vi "Node Main Operation.vi"(8 "error in (no error)":errorcluster, 11 "Node Actor in":refnum<class "Node Actor.lvclass">) -> (0 "error out":errorcluster, 3 "Node Actor out":refnum<class "Node Actor.lvclass">)   [LabVIEW 2024, in "Node Actor.lvclass"]
uses:
  Node Actor.lvclass
  Message/Message.lvclass/Message.ctl
  Node Actor.lvclass/Node Actor.ctl
  Message/Public Data/Read CMD Type.vi
  Message/Message.lvclass
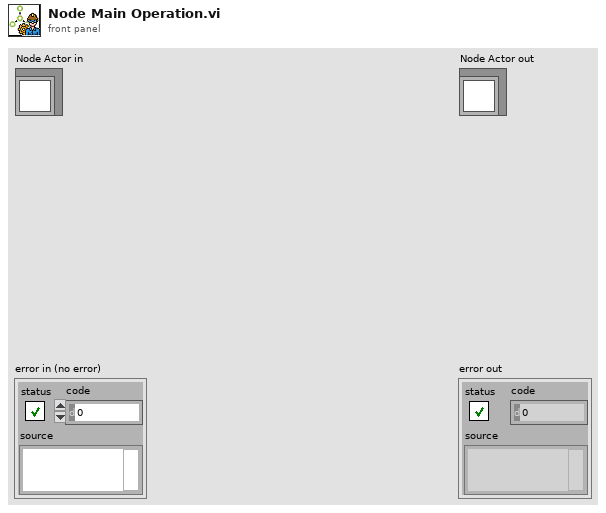
[diagram p1: front panel]
types:
  T1 = typedef "CMD Type.ctl" = enum16{"None", "General CMD", "1st CMD", "2nd CMD", "3rd CMD", "4th CMD", "5th CMD", "6th CMD", "7th CMD"}
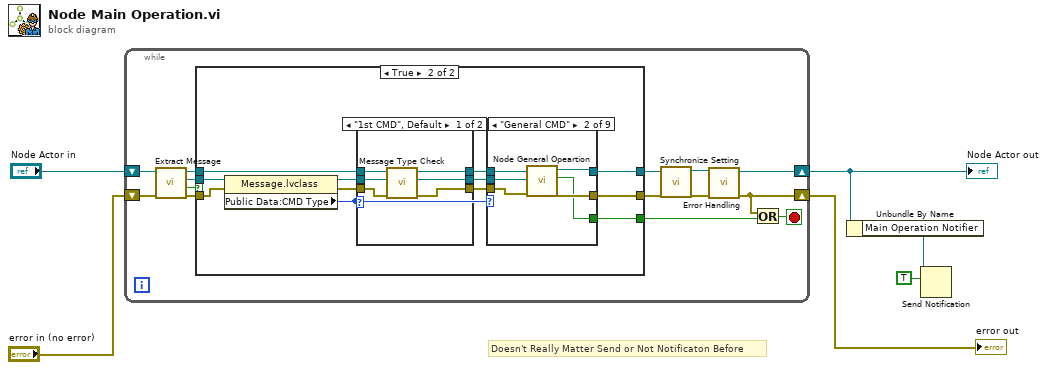
[diagram p0: block diagram]
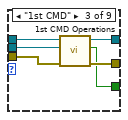
[diagram p5: hidden frame]
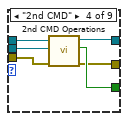
[diagram p6: hidden frame]
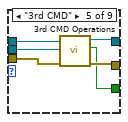
[diagram p7: hidden frame]
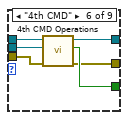
[diagram p8: hidden frame]
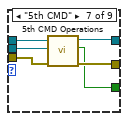
[diagram p9: hidden frame]
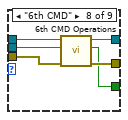
[diagram p10: hidden frame]
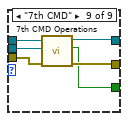
[diagram p11: hidden frame]
diagram:
  # "Doesn't Really Matter Send or Not Notificaton Before"
  n1 = while {
    shift-right: [w12] -> w1
    shift-left: "Node Actor in" -> [w19]
    shift-right: [w11] -> w4
    shift-left: "error in (no error)" -> [w18]
    stop <- w20 stop-if-true
    n2 = call-dynamic "Extract Message.vi"("error in (no error)"=w18, "Node Actor in"=w19) -> ("error out"=w15:errorcluster, "Valid"=w13:bool, "Message Out"=w16:refnum<class "Message.lvclass">, "Node Actor out"=w17:refnum<class "Node Actor.lvclass">)  [unwired: 6 in]
    n3 = case shown="True" w13 {
      tunnel: [w21 w34] -> w8
      tunnel: w17 -> [w22 w26]
      tunnel: w16 -> [_ w31]
      tunnel: w15 -> [w21 w30]
      tunnel: [w22 w33] -> w10
      tunnel: [_ w32] -> w14
      frame False {
      }
      frame True {
        n4 = property class="Message.lvclass"(reference=w31, error in=w30) -> (reference out=w28:refnum<class "Message.lvclass">, error out=w27:errorcluster, "Public Data:CMD Type"=w29:T1)
        n5 = case shown="\"1st CMD\", Default" w29 {
          tunnel: w28 -> [w39 w42]
          tunnel: w27 -> [w38 w41]
          tunnel: w26 -> [w40 w43]
          tunnel: [w35 w43] -> w25
          tunnel: [w36 w42] -> w24
          tunnel: [w37 w41] -> w23
          frame "1st CMD", Default {
            n6 = call-dynamic "Message Type Check.vi"("error in (no error)"=w38, "Message In"=w39, "Node Actor in"=w40) -> ("error out"=w37:errorcluster, "Message Out"=w36:refnum<class "Message.lvclass">, "Node Actor out"=w35:refnum<class "Node Actor.lvclass">)  [unwired: 6 in]
          }
          frame "General CMD" {
          }
        }
        n7 = case shown="\"General CMD\"" w29 {
          tunnel: w24 -> [_ w50 w56 w59 w68 w74 w80 w86 w92]
          tunnel: w25 -> [w45 w51 w57 w63 w69 w75 w81 w87 w93]
          tunnel: [w45 w47 w53 w62 w65 w72 w77 w84 w89] -> w33
          tunnel: w23 -> [w44 w49 w55 w58 w67 w73 w79 w85 w91]
          tunnel: [w44 w48 w54 w60 w66 w70 w78 w83 w90] -> w34
          tunnel: [_ w46 w52 w61 w64 w71 w76 w82 w88] -> w32
          frame "None", Default {
          }
          frame "General CMD" {
            n8 = call-dynamic "Node General Opeartion.vi"("error in (no error)"=w49, "Message In"=w50, "Node Actor in"=w51) -> ("error out"=w48:errorcluster, "Stop"=w46:bool, "Node Actor out"=w47:refnum<class "Node Actor.lvclass">)  [unwired: 6 in]
          }
          frame "1st CMD" {
            n9 = call-dynamic "1st CMD Operations.vi"("error in (no error)"=w55, "Message In"=w56, "System Actor in"=w57) -> ("error out"=w54:errorcluster, "Stop"=w52:bool, "System Actor out"=w53:refnum<class "Node Actor.lvclass">)  [unwired: 6 in]
          }
          frame "2nd CMD" {
            n10 = call-dynamic "2nd CMD Operations.vi"("error in (no error)"=w58, "Message In"=w59, "System Actor in"=w63) -> ("error out"=w60:errorcluster, "Stop"=w61:bool, "System Actor out"=w62:refnum<class "Node Actor.lvclass">)  [unwired: 6 in]
          }
          frame "3rd CMD" {
            n11 = call-dynamic "3rd CMD Operations .vi"("error in (no error)"=w67, "Message In"=w68, "System Actor in"=w69) -> ("error out"=w66:errorcluster, "Stop"=w64:bool, "System Actor out"=w65:refnum<class "Node Actor.lvclass">)  [unwired: 6 in]
          }
          frame "4th CMD" {
            n12 = call-dynamic "4th CMD Operations.vi"("error in (no error)"=w73, "Message In"=w74, "System Actor in"=w75) -> ("error out"=w70:errorcluster, "Stop"=w71:bool, "System Actor out"=w72:refnum<class "Node Actor.lvclass">)  [unwired: 6 in]
          }
          frame "5th CMD" {
            n13 = call-dynamic "5th CMD Operations.vi"("error in (no error)"=w79, "Message In"=w80, "System Actor in"=w81) -> ("error out"=w78:errorcluster, "Stop"=w76:bool, "System Actor out"=w77:refnum<class "Node Actor.lvclass">)  [unwired: 6 in]
          }
          frame "6th CMD" {
            n14 = call-dynamic "6th CMD Operations .vi"("error in (no error)"=w85, "Message In"=w86, "System Actor in"=w87) -> ("error out"=w83:errorcluster, "Stop"=w82:bool, "System Actor out"=w84:refnum<class "Node Actor.lvclass">)  [unwired: 6 in]
          }
          frame "7th CMD" {
            n15 = call-dynamic "7th CMD Operations.vi"("error in (no error)"=w91, "Message In"=w92, "System Actor in"=w93) -> ("error out"=w90:errorcluster, "Stop"=w88:bool, "System Actor out"=w89:refnum<class "Node Actor.lvclass">)  [unwired: 6 in]
          }
        }
      }
    }
    n16 = call-dynamic "Synchronize Setting.vi"("error in (no error)"=w8, "Node Actor in"=w10) -> ("error out"=w7:errorcluster, "Node Actor out"=w9:refnum<class "Node Actor.lvclass">)  [unwired: 8 in]
    n17 = call-dynamic "Error Handling.vi"("error in (no error)"=w7, "System Actor in"=w9) -> ("error out"=w11:errorcluster, "System Actor out"=w12:refnum<class "Node Actor.lvclass">)  [unwired: 8 in]
    n18 = Or(x=w11, y=w14) -> (x .or. y?=w20:bool)
  }
  "error out" <- w4
  "Node Actor out" <- w1
  n19 = Unbundle By Name(w1) -> ("Main Operation Notifier"=w3:refnum<notifier>)
  n20 = Send Notification(notification=TRUE, notifier=w3) -> ()  [unwired: 1 in, 2 out]
